vi "Unflatten.vi"(8 "error in (no error)":errorcluster, 11 "Continuous in":refnum<class "Magnetic Field Oxford Continuous.lvclass">) -> (0 "error out":errorcluster, 3 "Continuous out":refnum<class "Magnetic Field Oxford Continuous.lvclass">)   [LabVIEW 2023, in "Magnetic Field Oxford Continuous.lvclass"]
uses:
  Magnetic Field Oxford Continuous.lvclass
  Magnetic Field Oxford Continuous.lvclass/Magnetic Field Oxford Continuous.ctl
  Global/File Locations.vi
  Scanner/Scanner.lvclass
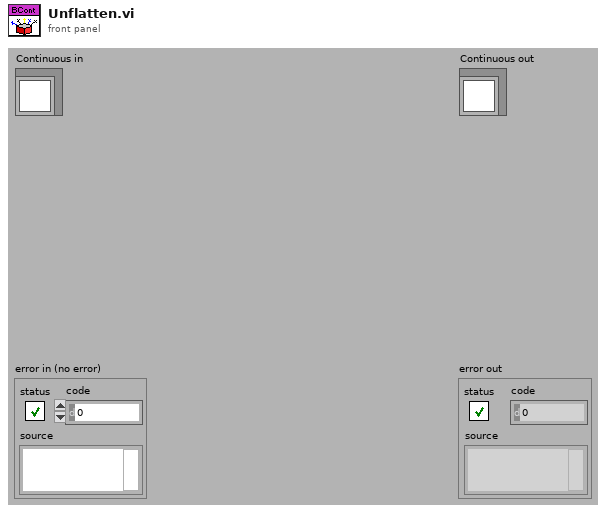
[diagram p1: front panel]
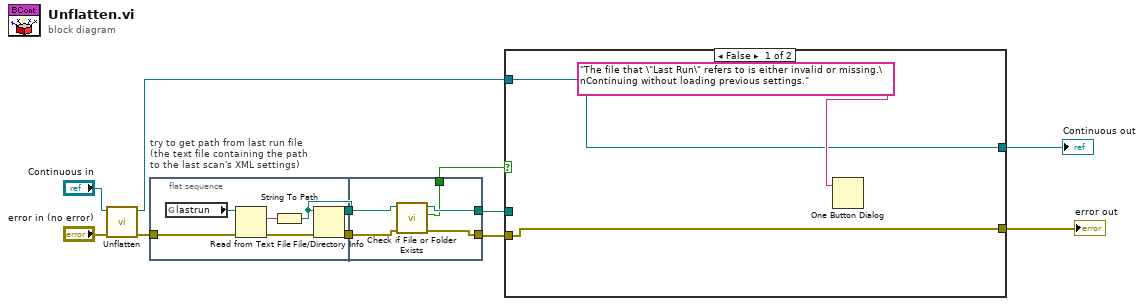
[diagram p0: block diagram]
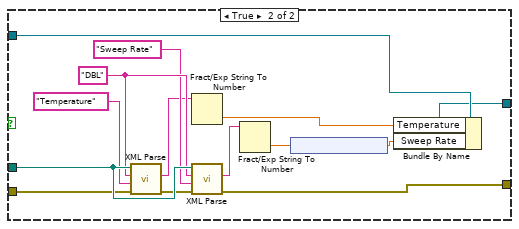
[diagram p2: hidden frame]
diagram:
  n1 = call-parent "Unflatten.vi"("error in (no error)"="error in (no error)", "Scanner in"="Continuous in") -> ("error out"=w8:errorcluster, "Scanner out"=w11:refnum<class "Magnetic Field Oxford Continuous.lvclass">)  [unwired: 8 in]
  n2 = flat-sequence "try to get path from last run file\n(the text file containing the path\nto the last scan's XML settings)" {
    tunnel: w8 -> [w12]
    tunnel: [w17] -> w3
    tunnel: [w13] -> w2
    tunnel: [w21] -> w5
    tunnel: [w22] -> w6
    tunnel: w3 -> [w19]
    tunnel: w2 -> [w18]
    tunnel: [w20] -> w1
    frame #0 {
      n3 = global read "File Locations.vi" "lastrun"() -> (w15:path)
      n4 = Read from Text File(file (use dialog)=w15, error in=w12) -> (text=w16:string, error out=w14:errorcluster)  [unwired: 4 out]
      n5 = String To Path(string=w16) -> (path=w17:path)
      n6 = File/Directory Info(path=w17, error in=w14) -> (error out=w13:errorcluster)  [unwired: 6 out]
    }
    frame #1 {
      n7 = call <vilib>:"Check if File or Folder Exists.vi"("error in (no error)"=w18, "path"=w19) -> ("error out"=w21:errorcluster, "file or folder exists?"=w20:bool, "dup path"=w22:path)  [unwired: 7 in]
    }
  }
  n8 = case shown="False" w1 {
    tunnel: w11 -> [w24 w39]
    tunnel: [w24 w38] -> w7
    tunnel: w6 -> [_ w37]
    tunnel: w5 -> [w23 w33]
    tunnel: [w23 w31] -> w4
    frame False {
      n9 = One Button Dialog(message="The file that \"Last Run\" refers to is either invalid or missing.\nContinuing without loading previous settings.") -> ()  [unwired: 1 in, 1 out]
    }
    frame True {
      w36 = "DBL"
      n10 = call "XML Parse.vi"("error in (no error)"=w33, "Name String"="Temperature", "Type String"=w36, "Path"=w37) -> ("error out"=w32:errorcluster, "String Out"=w30:string)  [unwired: 6 in]
      n11 = Fract/Exp String To Number(string=w30) -> (number=w27:dbl)  [unwired: 3 in, 1 out]
      n12 = call "XML Parse.vi"("error in (no error)"=w32, "Name String"="Sweep Rate", "Type String"=w36, "Path"=w37) -> ("error out"=w31:errorcluster, "String Out"=w29:string)  [unwired: 6 in]
      n13 = Fract/Exp String To Number(string=w29) -> (number=w28:dbl)  [unwired: 3 in, 1 out]
      n14 = node(w28) -> (w26:dbl[unit])
      n15 = Bundle By Name(cluster=w39, "Temperature"=w27, "Sweep Rate"=w26) -> (w38:refnum<class "Magnetic Field Oxford Continuous.lvclass">)
    }
  }
  "error out" <- w4
  "Continuous out" <- w7
